vi "i_n__v1.vi"(9 "d[n]":ext, 10 "ƒÆ[n-1]":ext, 11 "i[n-1]":ext) -> (3 "i[n]":ext)   [LabVIEW 2020]
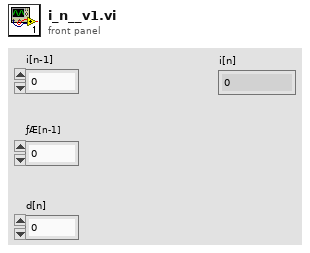
[diagram p1: front panel]
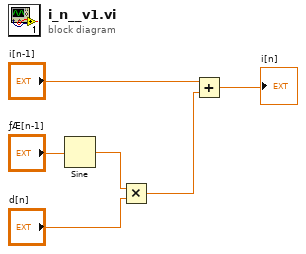
[diagram p0: block diagram]
diagram:
  n1 = Sine(x="ƒÆ[n-1]") -> (sin(x)=w5:ext)
  n2 = Multiply(x=w5, y="d[n]") -> (x*y=w2:ext)
  n3 = Add(x="i[n-1]", y=w2) -> (x+y=→"i[n]":ext)
